vi "Mouse Move.vi"() -> ()   [LabVIEW 2021]
uses:
  <vilib>/Utility/miscctls.llb/LVPoint32TypeDef.ctl
  <vilib>/Utility/miscctls.llb/LVPositionTypeDef.ctl
  <vilib>/QSI/Animation Toolkit/Animation.lvlib
panel:
  out "In Panel 2":bool
  in  "Numeric":dbl
  out "In Panel":bool
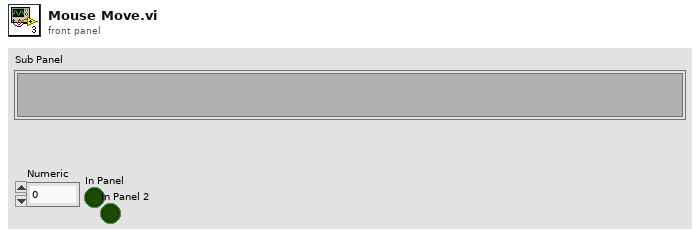
[diagram p1: front panel]
types:
  T1 = typedef "LVPositionTypeDef.ctl" = cluster{"Left":i32, "Top":i32}
  T2 = typedef "LVPoint32TypeDef.ctl" = cluster{"Horizontal":i32, "Vertical":i32}
  T3 = typedef "LVBoundsTypeDef.ctl" = cluster{"Width":u32, "Height":u32}
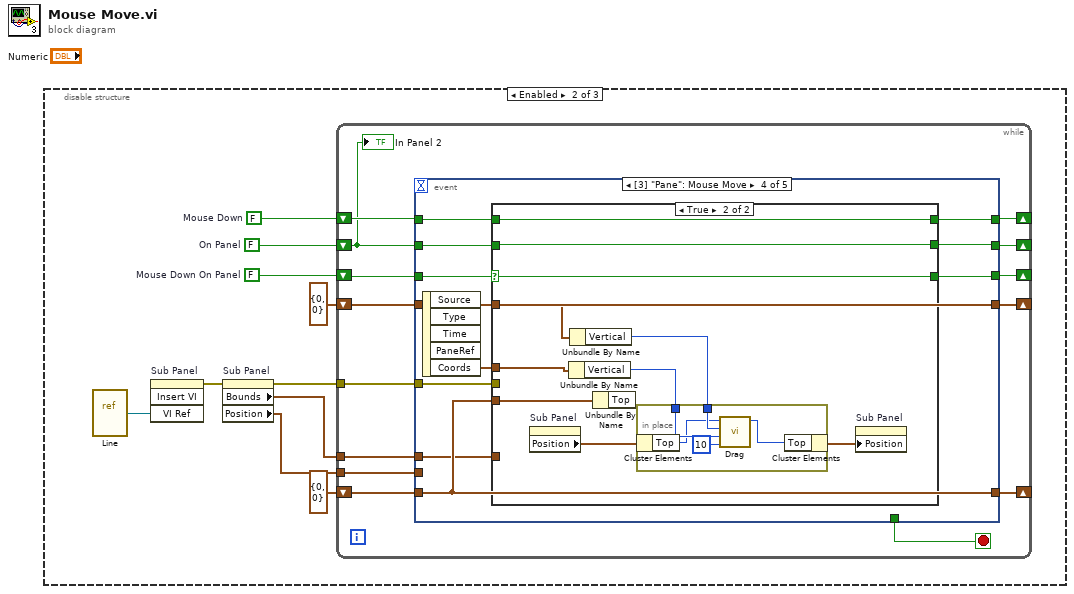
[diagram p0: block diagram]
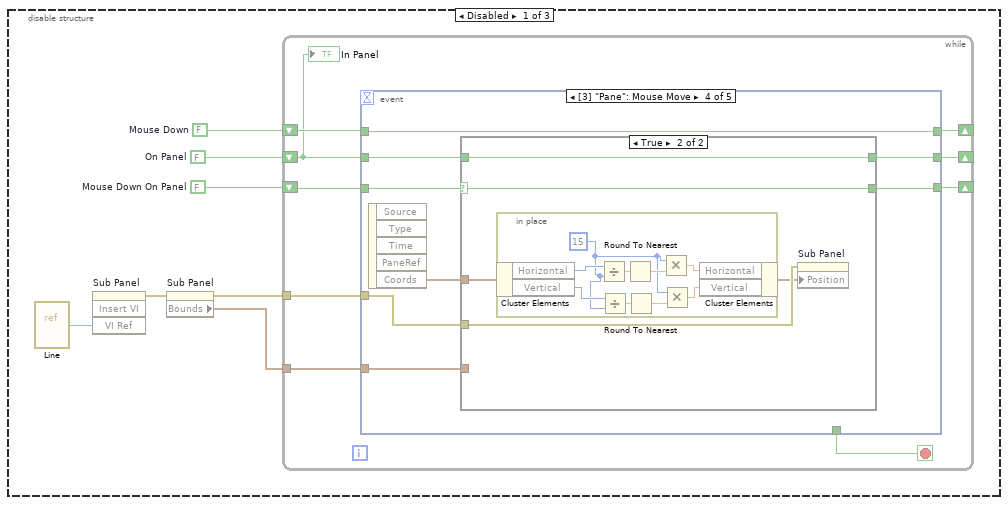
[diagram p2: hidden frame]
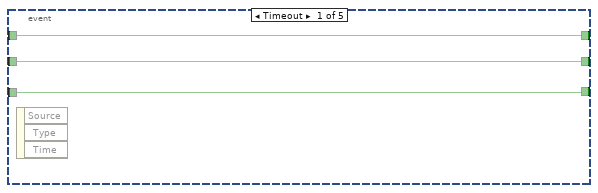
[diagram p3: hidden frame]
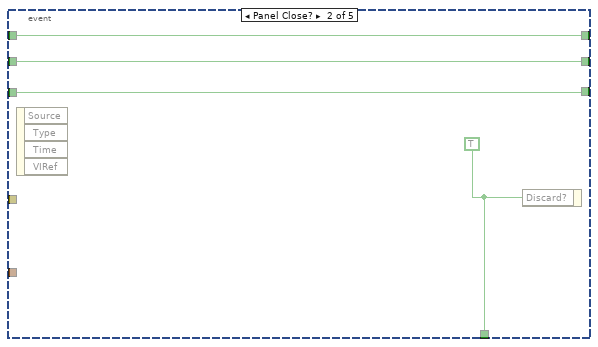
[diagram p4: hidden frame]
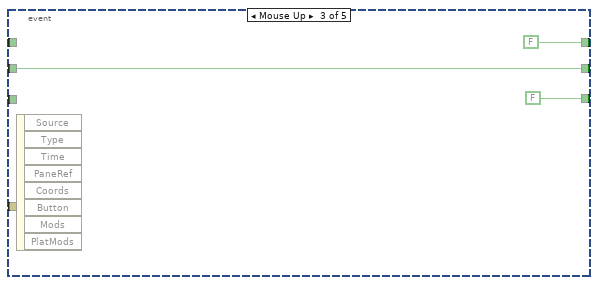
[diagram p5: hidden frame]
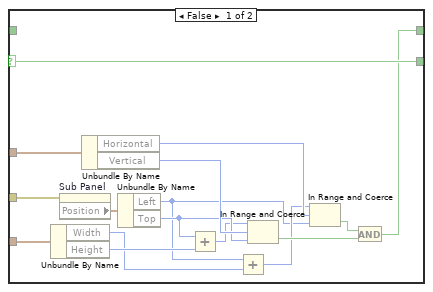
[diagram p6: hidden frame]
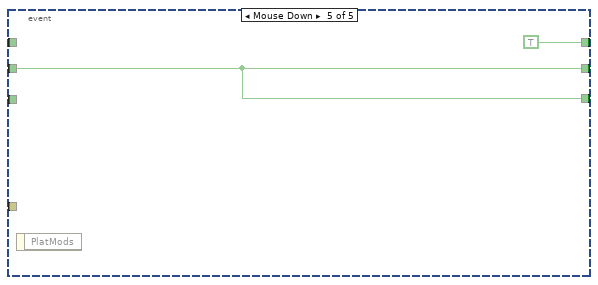
[diagram p7: hidden frame]
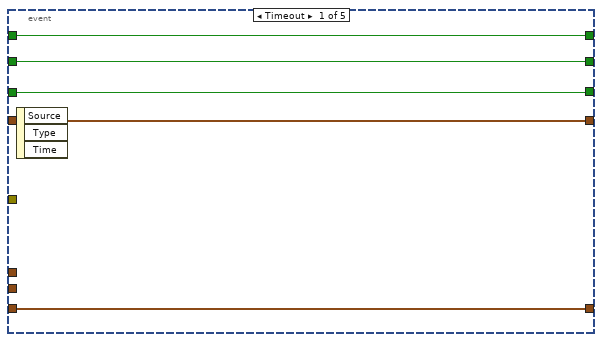
[diagram p8: hidden frame]
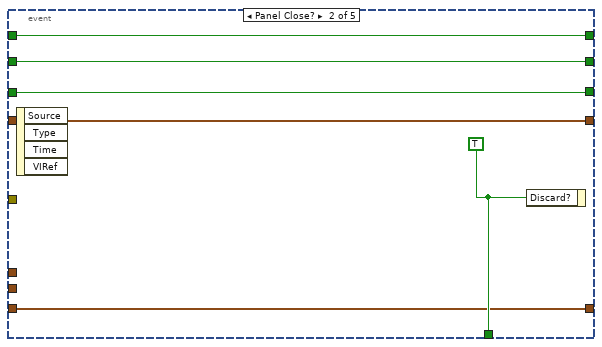
[diagram p9: hidden frame]
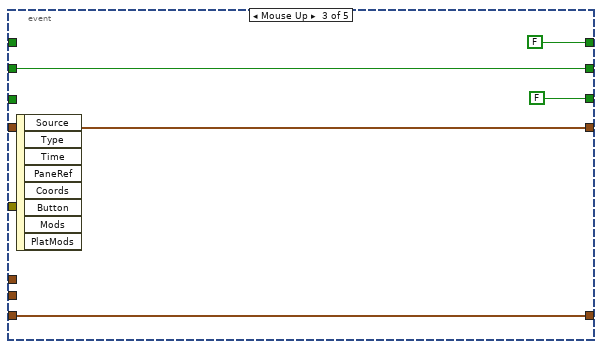
[diagram p10: hidden frame]
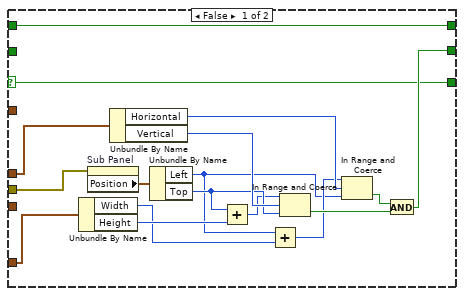
[diagram p11: hidden frame]
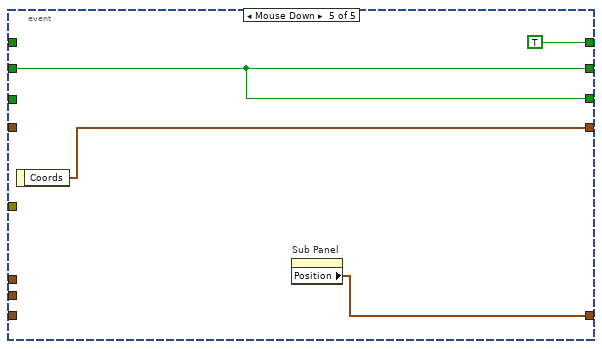
[diagram p12: hidden frame]
diagram:
  n1 = disable-structure shown="Enabled" {
    frame Disabled {
      w1 = FALSE  # Mouse Down On Panel
      w2 = FALSE  # On Panel
      w4 = FALSE  # Mouse Down
      n2 = vi-ref "Line.vi"() -> (w7:refnum<vi>)
      n3 = invoke on="Sub Panel" class="SubPnl" method="Insert VI"("VI Ref"=w7) -> (error out=w6:errorcluster)  [unwired: 3 in, 3 out]
      n4 = property on="Sub Panel" class="SubPnl"(error in=w6) -> (error out=w5:errorcluster, "Bounds"=w3:T3)  [unwired: 1 in, 1 out]
      n5 = while {
        tunnel: w5 -> [w12]
        shift-right: [w14] -> _
        shift-left: w4 -> [w15]
        tunnel: w3 -> [w13]
        shift-right: [w11] -> _
        shift-left: w2 -> [w10]
        shift-right: [w9] -> _
        shift-left: w1 -> [w8]
        stop <- w16 stop-if-true
        n6 = event shown="[3] \"Pane\": Mouse Move" {
          selector: _ -> [_ _ _ _ _]
          dyn-events: _ -> [_ _ _ _ _]
          timeout: _ -> [_ _ _ _ _]
          tunnel: [_ w23 _ _ _] -> w16
          tunnel: w15 -> [w19 w22 _ w34 _]
          tunnel: [w19 w22 FALSE ("Mouse Down") w34 TRUE ("Mouse Down")] -> w14
          tunnel: w13 -> [_ _ _ w32 _]
          tunnel: w10 -> [w18 w21 w25 w30 w65]
          tunnel: w12 -> [_ _ _ w33 _]
          tunnel: [w18 w21 w25 w27 w65] -> w11
          tunnel: [w17 w20 FALSE ("On Panel") w28 w65] -> w9
          tunnel: w8 -> [w17 w20 _ w29 _]
          event Timeout {
            n7 = event-data() -> ()  [unwired: 1 in, 3 out]
          }
          event Panel Close? {
            w23 = TRUE ("Discard?")
            n8 = event-data() -> ()  [unwired: 1 in, 4 out]
            n9 = event-data("Discard?"=w23) -> ()  [unwired: 1 in, 1 out]
          }
          event Mouse Up {
            n10 = event-data() -> ()  [unwired: 1 in, 8 out]
          }
          event Mouse Move {
            n11 = event-data() -> ("Coords"=w31:T2)  [unwired: 1 in, 4 out]
            n12 = case shown="True" w29 {
              selector: w29 -> [w36 w54]
              tunnel: w33 -> [w50 w55]
              tunnel: w32 -> [w49 _]
              tunnel: w31 -> [w47 w52]
              tunnel: w30 -> [_ w53]
              tunnel: [w36 w54] -> w28
              tunnel: [w35 w53] -> w27
              frame False {
                n13 = Unbundle By Name(w49) -> ("Width"=w45:u32, "Height"=w46:u32)
                n14 = property on="Sub Panel" class="SubPnl"(error in=w50) -> ("Position"=w48:T1)  [unwired: 1 in, 2 out]
                n15 = Unbundle By Name(w47) -> ("Horizontal"=w43:i32, "Vertical"=w44:i32)
                n16 = Unbundle By Name(w48) -> ("Left"=w37:i32, "Top"=w40:i32)
                n17 = Add(x=w40, y=w46) -> (x+y=w39:u32)
                n18 = Add(x=w37, y=w45) -> (x+y=w38:u32)
                n19 = In Range and Coerce(upper limit=w39, x=w44, lower limit=w40) -> (In Range?=w41:bool)  [unwired: 1 out]
                n20 = In Range and Coerce(upper limit=w38, x=w43, lower limit=w37) -> (In Range?=w42:bool)  [unwired: 1 out]
                n21 = And(x=w42, y=w41) -> (x .and. y?=w35:bool)
              }
              frame True {
                n22 = in-place {
                  w57 = 15 ("y")
                  n23 = in-place-cluster #1(w52) -> ("Horizontal"=w63:i32, "Vertical"=w58:i32)
                  n24 = Divide(x=w63, y=w57) -> (x/y=w64:dbl)
                  n25 = Divide(x=w58, y=w57) -> (x/y=w59:dbl)
                  n26 = Round To Nearest(number=w64) -> (nearest integer value=w62:dbl)
                  n27 = Round To Nearest(number=w59) -> (nearest integer value=w60:dbl)
                  n28 = Multiply(x=w57, y=w62) -> (x*y=w61:dbl)
                  n29 = Multiply(x=w57, y=w60) -> (x*y=w56:dbl)
                  n30 = in-place-cluster #1("Horizontal"=w61, "Vertical"=w56) -> (w51:T2)
                }
                n31 = property on="Sub Panel" class="SubPnl"(error in=w55, "Position"=w51) -> ()  [unwired: 1 in, 2 out]
              }
            }
          }
          event Mouse Down {
            n32 = event-data() -> ()  [unwired: 1 in, 1 out]
          }
        }
        "In Panel" <- w10
      }
    }
    frame Enabled {
      w70 = FALSE  # Mouse Down On Panel
      w71 = FALSE  # On Panel
      w73 = FALSE  # Mouse Down
      n33 = vi-ref "Line.vi"() -> (w76:refnum<vi>)
      n34 = invoke on="Sub Panel" class="SubPnl" method="Insert VI"("VI Ref"=w76) -> (error out=w75:errorcluster)  [unwired: 3 in, 3 out]
      n35 = property on="Sub Panel" class="SubPnl"(error in=w75) -> (error out=w74:errorcluster, "Bounds"=w72:T3, "Position"=w69:T1)  [unwired: 1 in, 1 out]
      n36 = while {
        tunnel: w74 -> [w86]
        shift-right: [w88] -> _
        shift-left: w73 -> [w89]
        tunnel: w72 -> [w87]
        shift-right: [w85] -> _
        shift-left: w71 -> [w84]
        shift-right: [w83] -> _
        shift-left: w70 -> [w82]
        tunnel: w69 -> [w81]
        shift-right: [w80] -> _
        shift-left: T2 {"Horizontal"=0, "Vertical"=0} ("Coords") -> [w79]
        shift-right: [w78] -> _
        shift-left: T1 {"Left"=0, "Top"=0} ("Position") -> [w77]
        stop <- w90 stop-if-true
        n37 = event shown="[3] \"Pane\": Mouse Move" {
          selector: _ -> [_ _ _ _ _]
          dyn-events: _ -> [_ _ _ _ _]
          timeout: _ -> [_ _ _ _ _]
          tunnel: [_ w101 _ _ _] -> w90
          tunnel: w89 -> [w95 w100 _ w109 _]
          tunnel: [w95 w100 FALSE ("Mouse Down") w108 TRUE ("Mouse Down")] -> w88
          tunnel: w87 -> [_ _ _ w112 _]
          tunnel: w84 -> [w94 w99 w105 w113 w152]
          tunnel: w86 -> [_ _ _ w111 _]
          tunnel: [w94 w99 w105 w110 w152] -> w85
          tunnel: [w93 w98 FALSE ("On Panel") w107 w152] -> w83
          tunnel: w82 -> [w93 w98 _ w114 _]
          tunnel: w81 -> [_ _ _ _ _]
          tunnel: [w92 w97 w103 w116 w151] -> w80
          tunnel: w79 -> [w92 w97 w103 w116 _]
          tunnel: [w91 w96 w102 w115 w150] -> w78
          tunnel: w77 -> [w91 w96 w102 w115 _]
          event Timeout {
            n38 = event-data() -> ()  [unwired: 1 in, 3 out]
          }
          event Panel Close? {
            w101 = TRUE ("Discard?")
            n39 = event-data() -> ()  [unwired: 1 in, 4 out]
            n40 = event-data("Discard?"=w101) -> ()  [unwired: 1 in, 1 out]
          }
          event Mouse Up {
            n41 = event-data() -> ()  [unwired: 1 in, 8 out]
          }
          event Mouse Move {
            n42 = event-data() -> ("Coords"=w117:T2)  [unwired: 1 in, 4 out]
            n43 = case shown="True" w114 {
              selector: w114 -> [w118 w139]
              tunnel: w117 -> [w123 w144]
              tunnel: w116 -> [_ w143]
              tunnel: w115 -> [_ w142]
              tunnel: w112 -> [w122 _]
              tunnel: w111 -> [w121 _]
              tunnel: [w120 w141] -> w110
              tunnel: w113 -> [_ w141]
              tunnel: w109 -> [w119 w140]
              tunnel: [w119 w140] -> w108
              tunnel: [w118 w139] -> w107
              frame False {
                n44 = Unbundle By Name(w122) -> ("Width"=w132:u32, "Height"=w133:u32)
                n45 = property on="Sub Panel" class="SubPnl"(error in=w121) -> ("Position"=w134:T1)  [unwired: 1 in, 2 out]
                n46 = Unbundle By Name(w123) -> ("Horizontal"=w130:i32, "Vertical"=w131:i32)
                n47 = Unbundle By Name(w134) -> ("Left"=w124:i32, "Top"=w127:i32)
                n48 = Add(x=w127, y=w133) -> (x+y=w126:u32)
                n49 = Add(x=w124, y=w132) -> (x+y=w125:u32)
                n50 = In Range and Coerce(upper limit=w126, x=w131, lower limit=w127) -> (In Range?=w128:bool)  [unwired: 1 out]
                n51 = In Range and Coerce(upper limit=w125, x=w130, lower limit=w124) -> (In Range?=w129:bool)  [unwired: 1 out]
                n52 = And(x=w129, y=w128) -> (x .and. y?=w120:bool)
              }
              frame True {
                n53 = property on="Sub Panel" class="SubPnl"() -> ("Position"=w138:T1)  [unwired: 2 in, 2 out]
                n54 = Unbundle By Name(w144) -> ("Vertical"=w136:i32)
                n55 = Unbundle By Name(w143) -> ("Vertical"=w135:i32)
                n56 = Unbundle By Name(w142) -> ()  [unwired: 1 out]
                n57 = in-place {
                  in-place-border: w136 -> [w148]
                  in-place-border: w135 -> [w147]
                  n58 = in-place-cluster #2(w138) -> ("Top"=w146:i32)
                  n59 = call <vilib>:"Drag.vi"("Extent"=10, "Current Mouse Position"=w148, "Start Mouse Position"=w147, "Start Drag Position"=w146) -> ("New Position"=w145:i32)  [unwired: 7 in]
                  n60 = in-place-cluster #2("Top"=w145) -> (w137:T1)
                }
                n61 = property on="Sub Panel" class="SubPnl"("Position"=w137) -> ()  [unwired: 2 in, 2 out]
              }
            }
          }
          event Mouse Down {
            n62 = event-data() -> ("Coords"=w151:T2)  [unwired: 1 in]
            n63 = property on="Sub Panel" class="SubPnl"() -> ("Position"=w150:T1)  [unwired: 2 in, 2 out]
          }
        }
        "In Panel 2" <- w84
      }
    }
    frame Disabled {
    }
  }
